vi "Initialize From File.vi"(0 "Commit in":refnum<class "Commit.lvclass">, 11 "error in (no error)":errorcluster) -> (4 "Commit out":refnum<class "Commit.lvclass">, 15 "error out":errorcluster)   [LabVIEW 2017, in "CL_G3_VIComponentBuilder.lvlib" / "Commit.lvclass"]
doc: "Initializes the class from the configuration file."
uses:
  Commit.lvclass
  Commit.lvclass/Commit.ctl
  Accessors/Read Commit Config File.vi
  Accessors/Write Exports Commit Destination Folder.vi
  <vilib>/Utility/config.llb/NI_LVConfig.lvlib
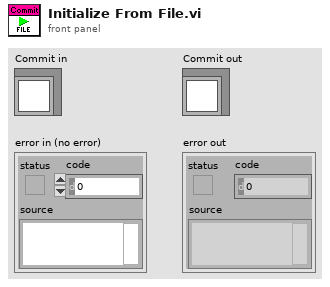
[diagram p1: front panel]
types:
  T1 = cluster{"Export's Commit Destination Folder":path}
  T2 = typedef "NI_LVConfig.lvlib/Config Data RefNum.ctl" = refnum<k1>
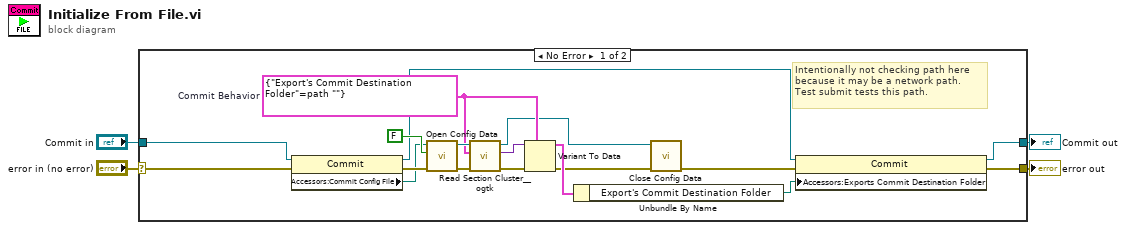
[diagram p0: block diagram]
diagram:
  n1 = case shown="No Error" "error in (no error)" {
    selector: "error in (no error)" -> [w9 w24]
    tunnel: [w8 w24] -> w3
    tunnel: [w10 w23] -> w1
    tunnel: "Commit in" -> [w13 w23]
    frame No Error {
      w19 = T1 {"Export's Commit Destination Folder"=path ""}  # Commit Behavior
      # "Intentionally not checking path here\nbecause it may be a network path. \nTest submit tests this path."
      n2 = property class="Commit"(reference=w13, error in=w9) -> (reference out=w12:refnum<class "Commit.lvclass">, error out=w15:errorcluster, "Accessors:Commit Config File"=w6:path)
      n3 = call <vilib>:"Open Config Data.vi"("error in (no error)"=w15, "create file if necessary (T)"=FALSE, "configuration file path"=w6) -> ("error out"=w17:errorcluster, "refnum"=w21:T2)  [unwired: 6 in, 1 out]
      n4 = call <userlib>:"Read Section Cluster__ogtk.vi"("error in (no error)"=w17, "Section Formatted Cluster Type"=w19, "refnum"=w21) -> ("error out"=w16:errorcluster, "Section Formatted Cluster"=w20:variant, "dup refnum"=w11:T2)  [unwired: 4 in, 2 out]
      n5 = Variant To Data(error in=w16, type=w19, Variant=w20) -> (data=w18:T1, error out=w14:errorcluster)
      n6 = Unbundle By Name(w18) -> ("Export's Commit Destination Folder"=w7:path)
      n7 = call <vilib>:"Close Config Data.vi"("error in (no error)"=w14, "refnum"=w11) -> ("error out"=w5:errorcluster)  [unwired: 8 in, 1 out]
      n8 = property class="Commit"(reference=w12, error in=w5, "Accessors:Exports Commit Destination Folder"=w7) -> (reference out=w10:refnum<class "Commit.lvclass">, error out=w8:errorcluster)
    }
    frame Error {
    }
  }
  "error out" <- w3
  "Commit out" <- w1
